vi "Settings Dialog.vi"(8 "error in (no error)":errorcluster, 11 "Settings in":T1) -> (0 "error out":errorcluster, 1 "Cancelled?":bool, 2 "UI Refresh Needed?":bool, 3 "Settings out":T1)   [LabVIEW 2014, in "Demonstrator Settings.lvlib"]
doc: "Dialog for selecting user specified settings."
uses:
  Demonstrator Settings.lvlib
  Settings.ctl
  Acquisition/Hardware Configuration.ctl
  Acquisition/Signal Type.ctl
  Logging/Logging Configuration.ctl
  <vilib>/Utility/xml.llb/Write to XML File(string).vi
  Acquisition/Demonstrator Acquisition.lvlib
  Logging/Demonstrator Logging.lvlib
panel:
  in  "Log File Path":path
  in  "Signal Type":u16(ring) items=["Sine Wave", "Square with Noise"]
  in  "Cancel Button":bool
  in  "OK Button":bool
  # "Non visible portion of dialog (needed for connector pane)."
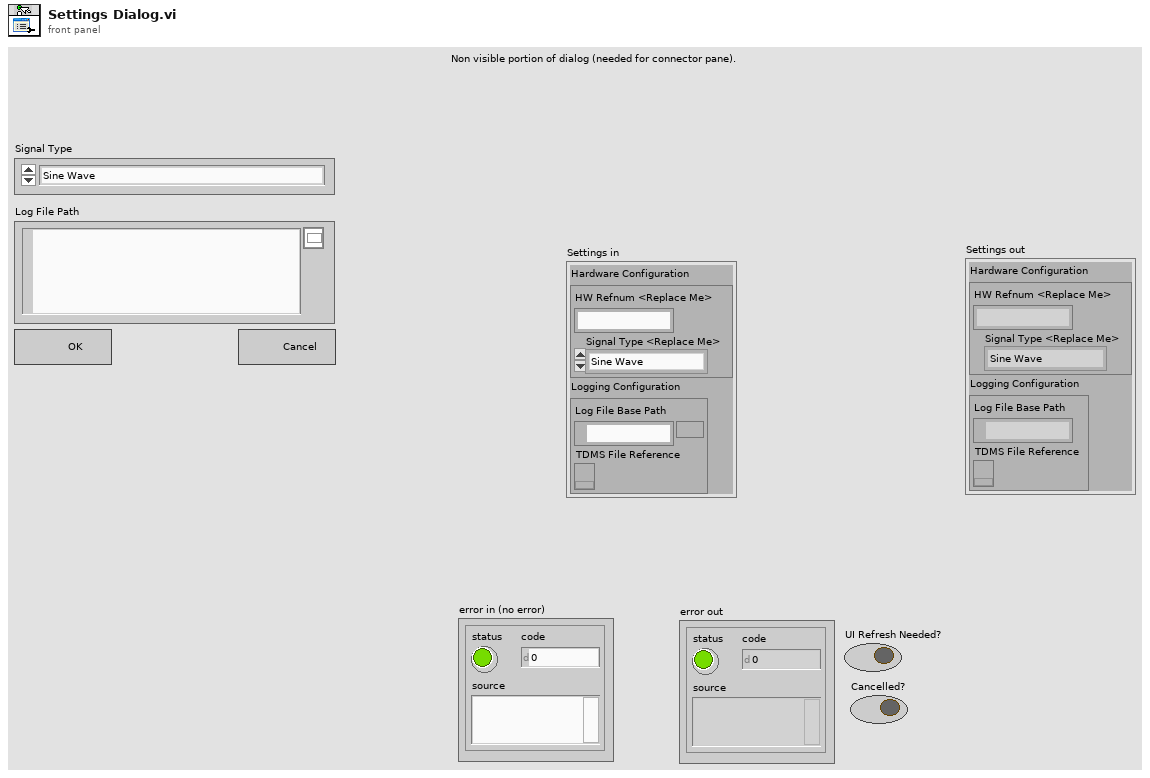
[diagram p1: front panel]
types:
  T1 = typedef "Demonstrator Settings.lvlib/Settings.ctl" = cluster{"Hardware Configuration":T2, "Logging Configuration":T4}
  T2 = typedef "Demonstrator Acquisition.lvlib/Hardware Configuration.ctl" = cluster{"HW Refnum <Replace Me>":string, "Signal Type <Replace Me>":T3}
  T3 = typedef "Demonstrator Acquisition.lvlib/Signal Type.ctl" = enum16{"Sine Wave", "Square with Noise"}
  T4 = typedef "Demonstrator Logging.lvlib/Logging Configuration.ctl" = cluster{"Log File Base Path":path, "TDMS File Reference":refnum<k34>}
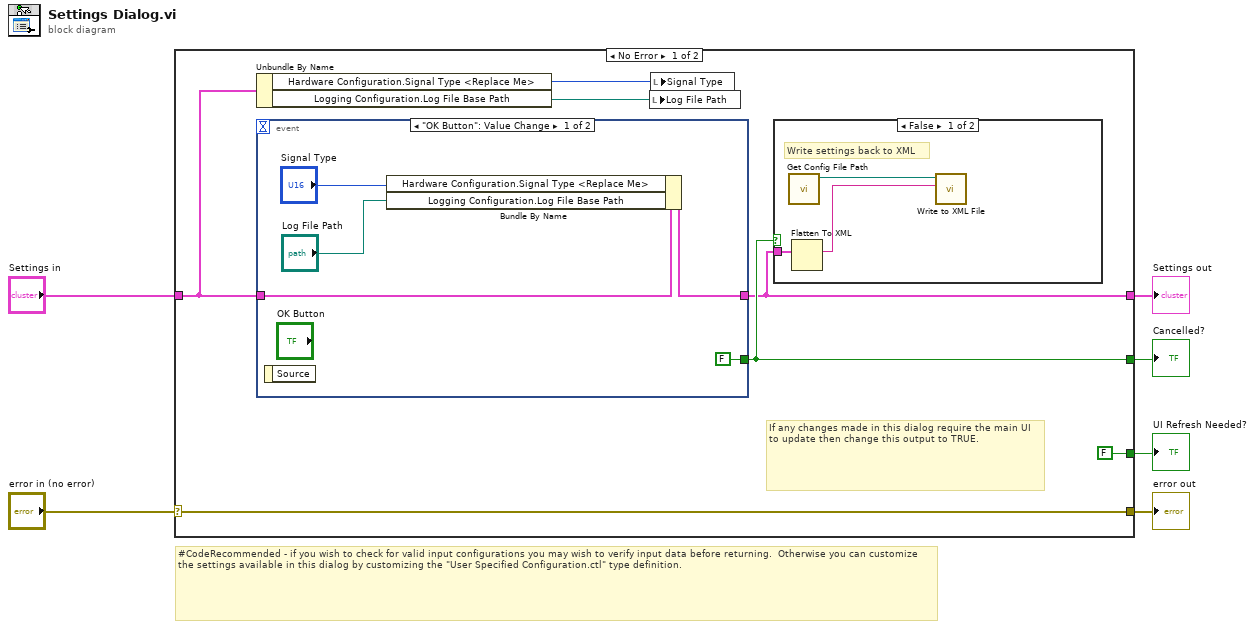
[diagram p0: block diagram]
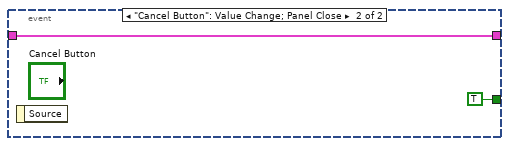
[diagram p3: hidden frame]
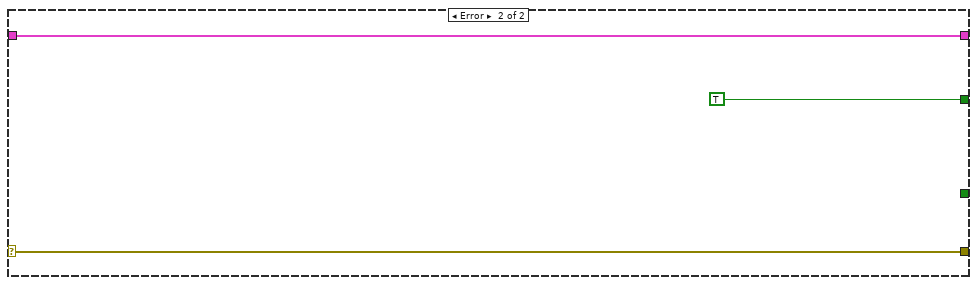
[diagram p4: hidden frame]
diagram:
  # "#CodeRecommended - if you wish to check for valid input configurations you may wish to verify input data before returning.  Otherwise you can customize the settings available in this dialog by customizing the \"User Specified Configuration.ctl\" type definition."
  n1 = case shown="No Error" "error in (no error)" {
    selector: "error in (no error)" -> [w13 w26]
    tunnel: [w13 w26] -> w5
    tunnel: "Settings in" -> [w9 w25]
    tunnel: [w10 w25] -> w3
    tunnel: [FALSE ("UI Refresh Needed?") _] -> w2
    tunnel: [w11 TRUE ("UI Refresh Needed?")] -> w1
    frame No Error {
      # "If any changes made in this dialog require the main UI to update then change this output to TRUE."
      n2 = Unbundle By Name(w9) -> ("Hardware Configuration.Signal Type <Replace Me>"=w8:T3, "Logging Configuration.Log File Base Path"=w7:path)
      n3 = event shown="[0] \"OK Button\": Value Change" {
        selector: _ -> [_ _]
        dyn-events: _ -> [_ _]
        timeout: _ -> [_ _]
        tunnel: [w19 w23] -> w10
        tunnel: w9 -> [w20 w23]
        tunnel: [FALSE ("UI Refresh Needed?") TRUE ("UI Refresh Needed?")] -> w11
        event "OK Button": Value Change {
          n4 = event-data() -> ()  [unwired: 1 in, 1 out]
          n5 = Bundle By Name(cluster=w20, "Hardware Configuration.Signal Type <Replace Me>"="Signal Type", "Logging Configuration.Log File Base Path"="Log File Path") -> (w19:T1)
        }
        event "Cancel Button": Value Change; Panel Close {
          n6 = event-data() -> ()  [unwired: 1 in, 1 out]
        }
      }
      n7 = local write "Log File Path"(w7) -> ()
      n8 = local write "Signal Type"(w8) -> ()
      n9 = case shown="False" w11 {
        tunnel: w10 -> [w15 _]
        frame False {
          # "Write settings back to XML"
          n10 = call "Get Config File Path.vi"() -> ("XML File Path"=w16:path)  [unwired: 10 in, 1 out]
          n11 = Flatten To XML(anything=w15) -> (xml string=w14:string)
          n12 = call-poly <vilib>:"Write to XML File.vi"("XML Input"=w14, "XML File Path"=w16) -> ()  [unwired: 7 in, 3 out]
        }
        frame True {
        }
      }
    }
    frame Error {
    }
  }
  "UI Refresh Needed?" <- w2
  "error out" <- w5
  "Settings out" <- w3
  "Cancelled?" <- w1
